vi "Check if Actuator is in Target position.vi"(8 "error in":errorcluster, 9 "Target":i16, 10 "Actuator name":string, 11 "UTP IO Session in":T1) -> (0 "error out":errorcluster, 2 "Target Position Reached?":bool, 3 "UTP IO Session out":T1)   [LabVIEW 2023, in "Actuators.lvlib"]
uses:
  <vilib>/Noffz/UTP IO/UTP IO Library/Typedefs/Session Handle.ctl
  <vilib>/Noffz/UTP IO/UTP IO Library/UTP IO Pool Session.lvclass
  <vilib>/Noffz/UTP IO/UTP IO Library/methods/poly/plc/Read PLC Variable (Boolean).vi
  Actuators.lvlib
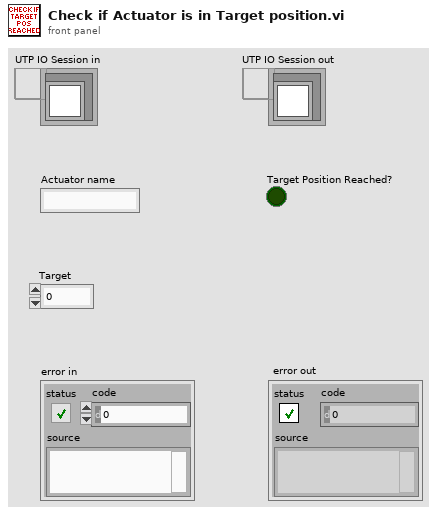
[diagram p1: front panel]
types:
  T1 = typedef "UTP IO Library.lvlib/UTP IO Pool Session.lvclass/Session Handle.ctl" = refnum<data-value>
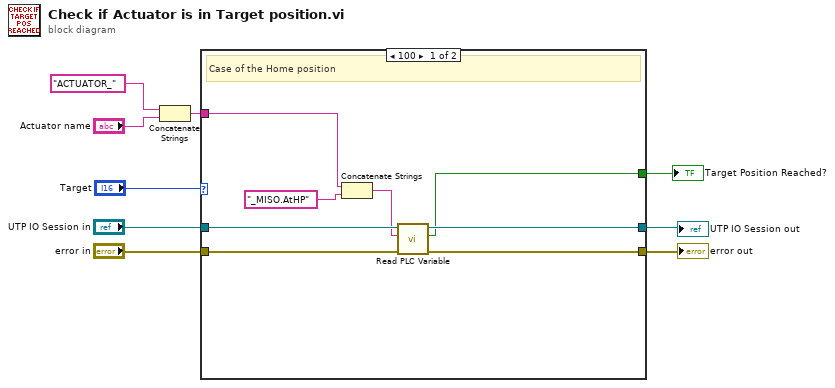
[diagram p0: block diagram]
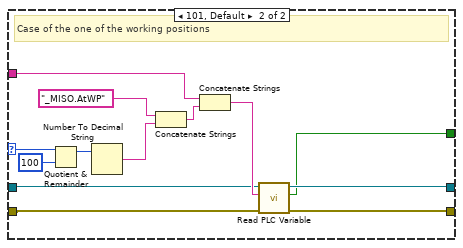
[diagram p2: hidden frame]
diagram:
  n1 = Concatenate Strings("ACTUATOR_" ("string"), "Actuator name") -> (w4:string)
  n2 = case shown="100" "Target" {
    selector: "Target" -> [_ w23]
    tunnel: "UTP IO Session in" -> [w17 w29]
    tunnel: "error in" -> [w16 w28]
    tunnel: w4 -> [w15 w27]
    tunnel: [w13 w26] -> w3
    tunnel: [w12 w25] -> w2
    tunnel: [w10 w18] -> w1
    frame 100 {
      # "Case of the Home position"
      n3 = Concatenate Strings(w15, "_MISO.AtHP" ("string")) -> (w14:string)
      n4 = call-poly <vilib>:"Read PLC Variable.vi"("error in (no error)"=w16, "variable name"=w14, "UTP IO Session in"=w17) -> ("error out"=w12:errorcluster, "value"=w10:bool, "UTP IO Session out"=w13:T1)  [unwired: 6 in]
    }
    frame 101, Default {
      # "Case of the one of the working positions"
      n5 = Quotient & Remainder(x=w23, y=i16 100) -> (x-y*floor(x/y)=w19:i16)  [unwired: 1 out]
      n6 = Number To Decimal String(number=w19) -> (decimal integer string=w21:string)  [unwired: 1 in]
      n7 = Concatenate Strings("_MISO.AtWP" ("string"), w21) -> (w20:string)
      n8 = Concatenate Strings(w27, w20) -> (w30:string)
      n9 = call-poly <vilib>:"Read PLC Variable.vi"("error in (no error)"=w28, "variable name"=w30, "UTP IO Session in"=w29) -> ("error out"=w25:errorcluster, "value"=w18:bool, "UTP IO Session out"=w26:T1)  [unwired: 6 in]
    }
  }
  "UTP IO Session out" <- w3
  "error out" <- w2
  "Target Position Reached?" <- w1
